vi "live page.vi"() -> ()   [LabVIEW 2019]
panel:
  in  "pellet detected View 2":T1(plugin-control)
  in  "Live View 2":T1(plugin-control)
  in  "average result array":dbl[](array[numeric])
  in  "live result array":dbl[](array[numeric])
  in  "Caption.Text":string
  in  "Tab Control":enum32{"LIVE VIEW", "Pellet Detected View"}(tab) caption="DISC 26"
  out "Live View":T1(plugin-control)
  out "pellet detected View":T1(plugin-control)
  out ">18 26a":dbl(slide)=1.0 caption=">18 mm" scale=0.0..100.0
  out "16-18 26a":dbl(slide)=1.0 caption="16-18 mm" scale=0.0..100.0
  out "12.5-16 a":dbl(slide)=1.0 caption="12.5-16 mm" scale=0.0..100.0
  out "9-12.5  a":dbl(slide)=1.0 caption="9-12.5 mm" scale=0.0..100.0
  out "6.3-9  a":dbl(slide)=1.0 caption="6.3-9 mm" scale=0.0..100.0
  out "5-6.3  a":dbl(slide)=1.0 caption="5-6.3 mm" scale=0.0..100.0
  out "<5  a":dbl(slide)=1.0 caption="<5 mm" scale=0.0..100.0
  out ">18":dbl(slide)=1.0 caption=">18 mm" scale=0.0..100.0
  out "16-18":dbl(slide)=1.0 caption="16-18 mm" scale=0.0..100.0
  out "12.5-16":dbl(slide)=1.0 caption="12.5-16 mm" scale=0.0..100.0
  out "9-12.5":dbl(slide)=1.0 caption="9-12.5 mm" scale=0.0..100.0
  out "6.3-9":dbl(slide)=1.0 caption="6.3-9 mm" scale=0.0..100.0
  out "5-6.3":dbl(slide)=1.0 caption="5-6.3 mm" scale=0.0..100.0
  out "<5":dbl(slide)=1.0 caption="<5 mm" scale=0.0..100.0
  # "Live Result"
  # "Average Result"
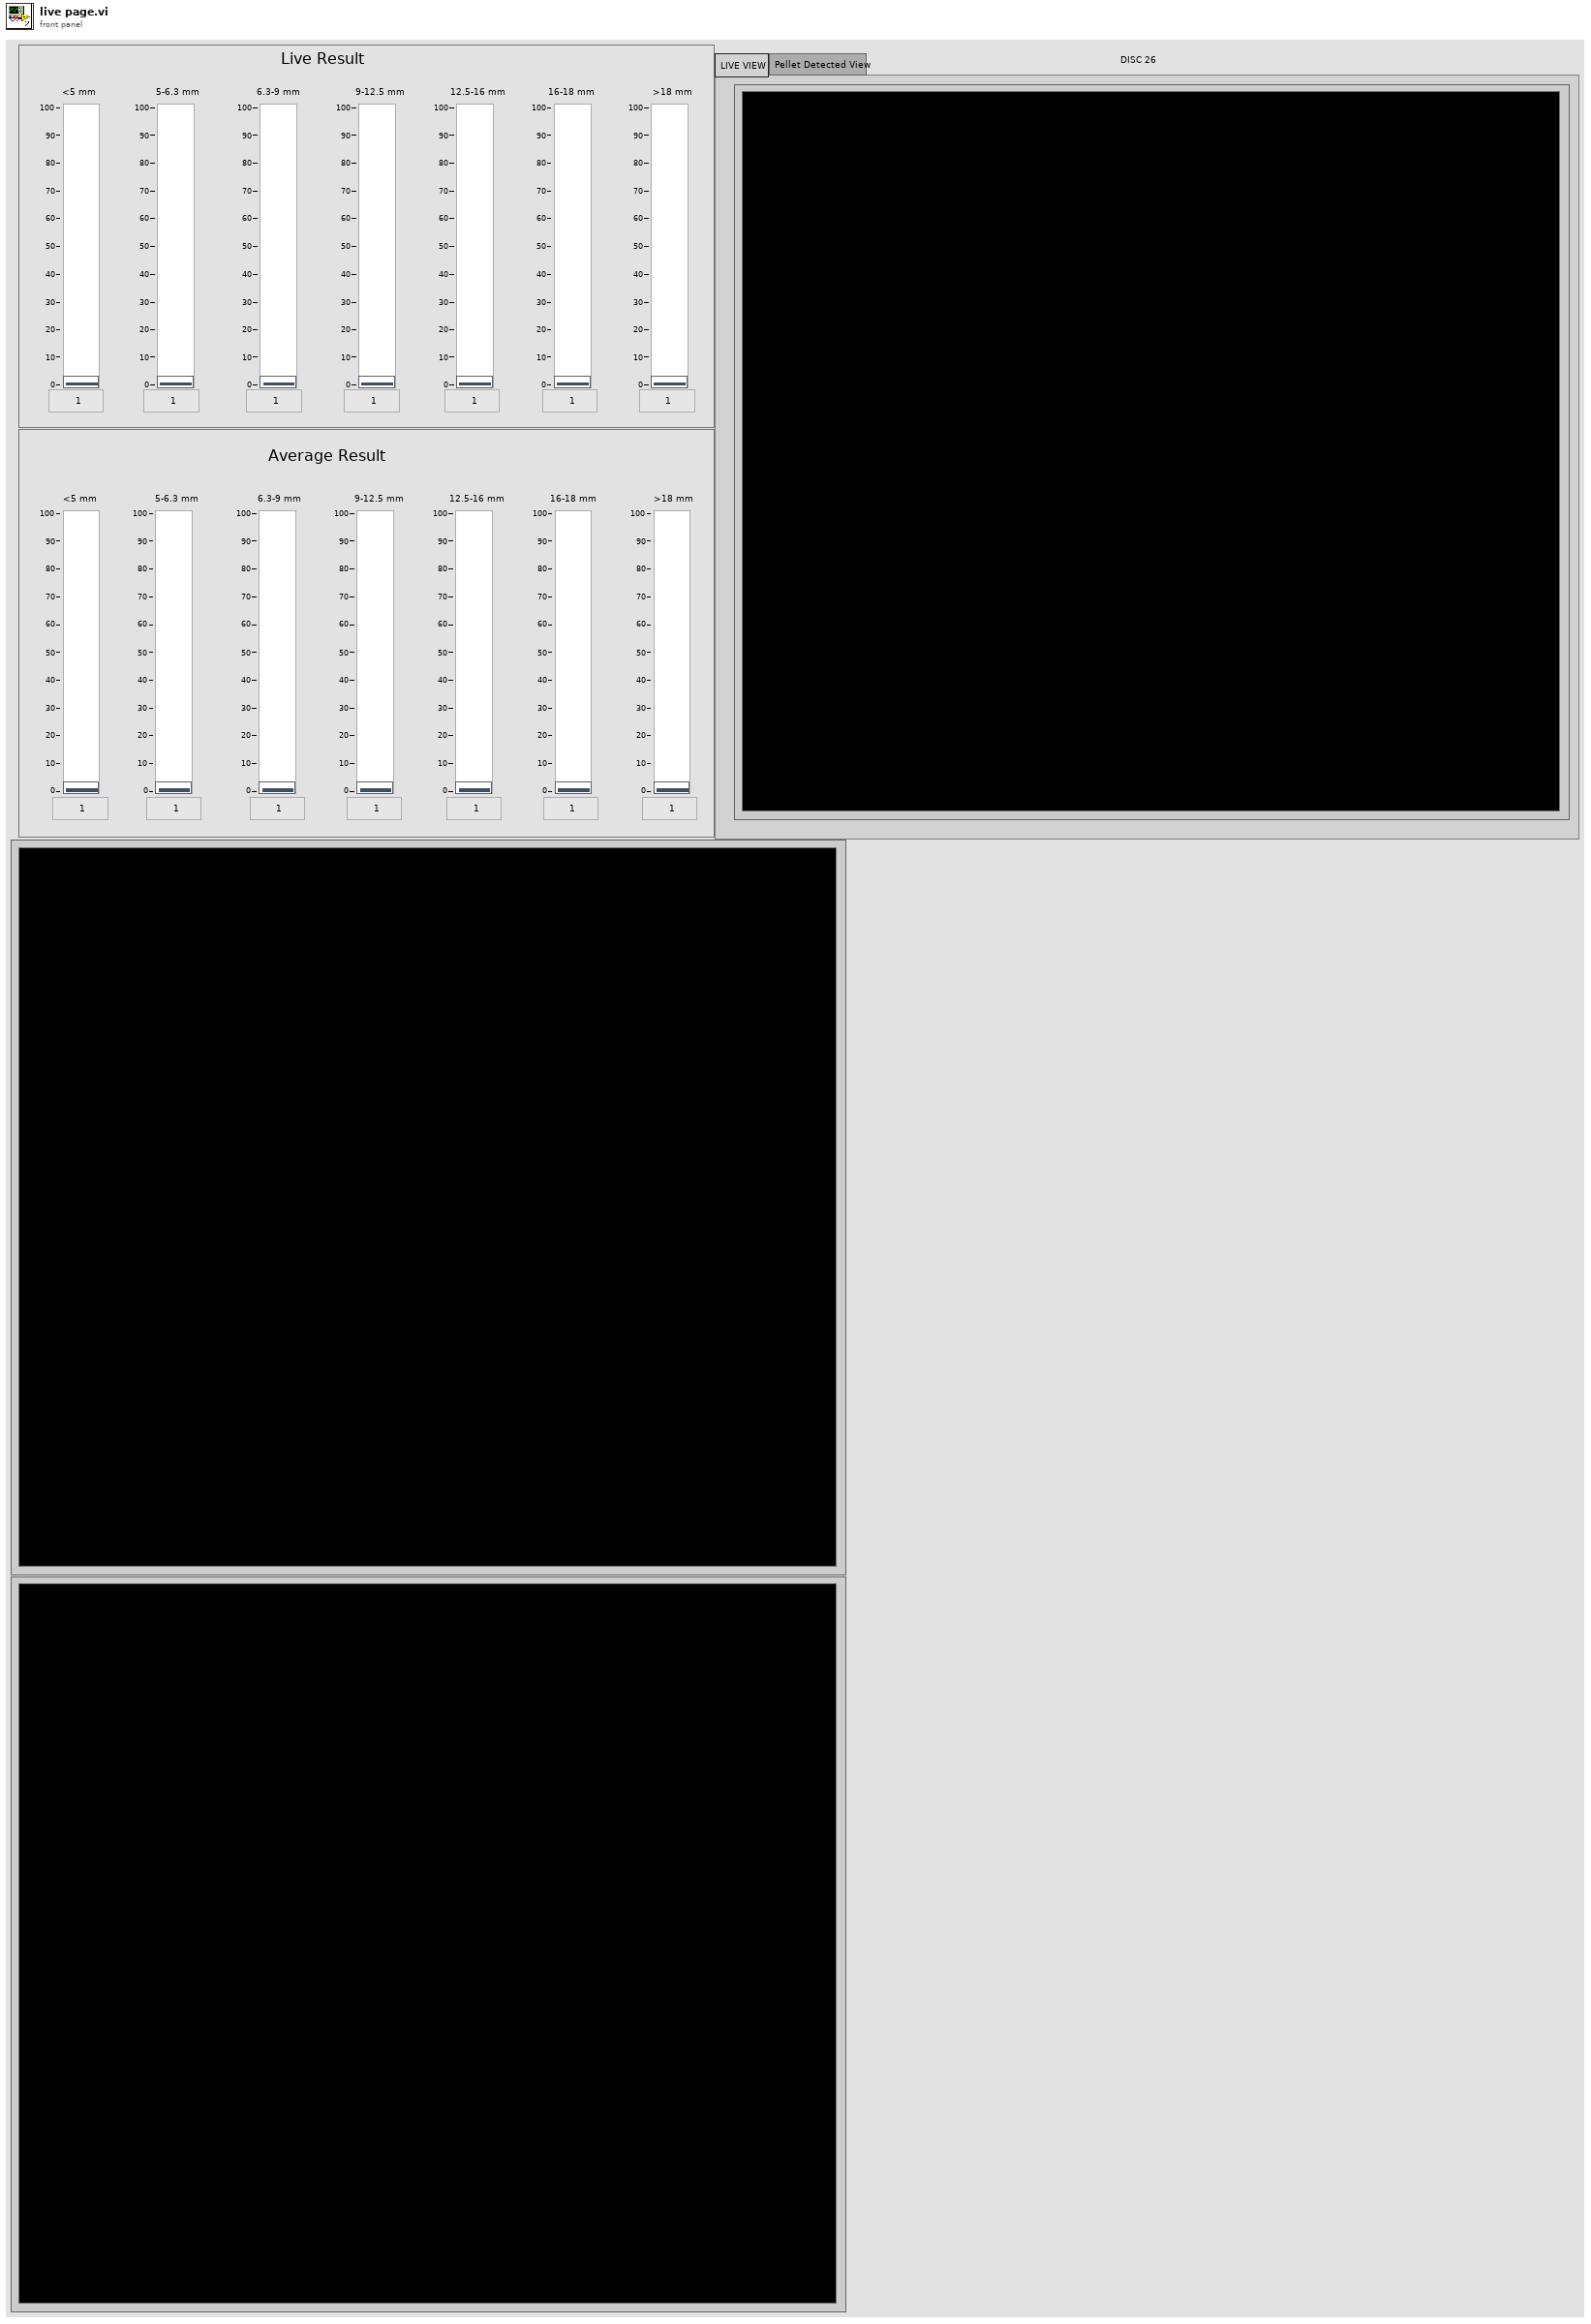
[diagram p1: front panel]
types:
  T1 = typedef "IMAQ Image.ctl" = refnum<image>
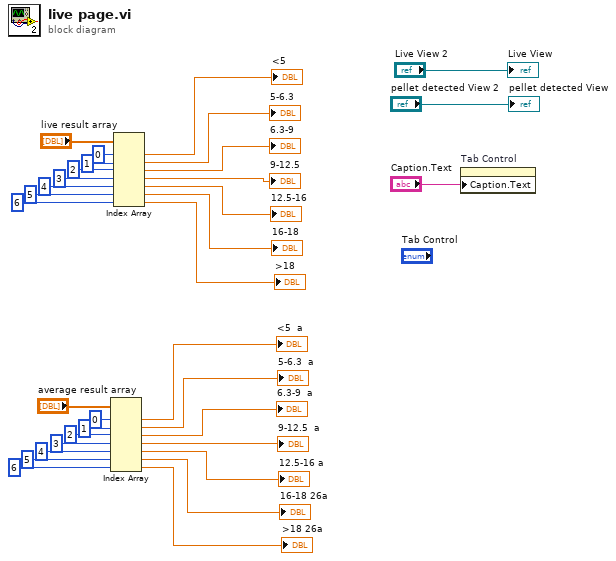
[diagram p0: block diagram]
diagram:
  n1 = Index Array(array="average result array", index #1=0 ("index"), index #2=1 ("index"), index #3=2 ("index"), index #4=3 ("index"), index #5=4 ("index"), index #6=5 ("index"), index #7=6 ("index")) -> (element #1=→"<5  a":dbl, element #2=→"5-6.3  a":dbl, element #3=→"6.3-9  a":dbl, element #4=→"9-12.5  a":dbl, element #5=→"12.5-16 a":dbl, element #6=→"16-18 26a":dbl, element #7=→">18 26a":dbl)
  n2 = Index Array(array="live result array", index #1=0 ("index"), index #2=1 ("index"), index #3=2 ("index"), index #4=3 ("index"), index #5=4 ("index"), index #6=5 ("index"), index #7=6 ("index")) -> (element #1=→"<5":dbl, element #2=→"5-6.3":dbl, element #3=→"6.3-9":dbl, element #4=→"9-12.5":dbl, element #5=→"12.5-16":dbl, element #6=→"16-18":dbl, element #7=→">18":dbl)
  n3 = property on="Tab Control" class="TabCtl (strict)"("Caption.Text"="Caption.Text") -> ()  [unwired: 2 in, 2 out]
  "Live View" <- "Live View 2"
  "pellet detected View" <- "pellet detected View 2"
